vi "Create AI Channel.vi"(6 "index":i32, 8 "error in":errorcluster, 9 "default value":dbl, 10 "name":string, 11 "AI channel in":refnum<class "AI Channel.lvclass">) -> (0 "error out":errorcluster, 3 "AI channel out":refnum<class "AI Channel.lvclass">)   [LabVIEW 2020, in "Scan Engine Scripting.lvlib" / "AI Channel.lvclass"]
uses:
  AI Channel.lvclass
  Channel/Type.ctl
  Channel/Channel.lvclass
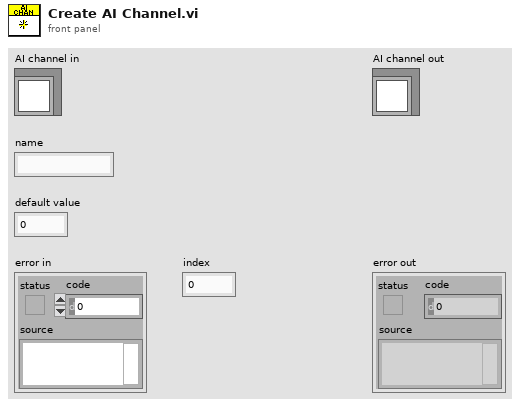
[diagram p1: front panel]
types:
  T1 = typedef "Scan Engine Scripting.lvlib/Channel.lvclass/Type.ctl" = enum16{"Input", "Output"}
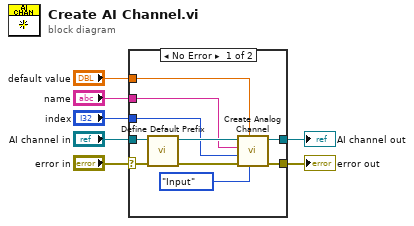
[diagram p0: block diagram]
diagram:
  n1 = case shown="No Error" "error in" {
    selector: "error in" -> [w16 w19]
    tunnel: [w13 w19] -> w6
    tunnel: [w12 w18] -> w4
    tunnel: "AI channel in" -> [w17 w18]
    tunnel: "name" -> [w9 _]
    tunnel: "default value" -> [w8 _]
    tunnel: "index" -> [w10 _]
    frame No Error {
      n2 = call-dynamic "Define Default Prefix.vi"("error in"=w16, "AI channel in"=w17) -> ("error out"=w15:errorcluster, "AI channel out"=w14:refnum<class "AI Channel.lvclass">)  [unwired: 8 in]
      n3 = call-dynamic "Create Analog Channel.vi"("type"=Type."Input", "default value"=w8, "error in"=w15, "index"=w10, "name"=w9, "analog channel in"=w14) -> ("error out"=w13:errorcluster, "analog channel out"=w12:refnum<class "AI Channel.lvclass">)  [unwired: 4 in]
    }
    frame Error {
    }
  }
  "error out" <- w6
  "AI channel out" <- w4
